vi "coag model linear regression.vi"(4 "averaged data":T1, 6 "all coag in":dbl[](array[numeric]), 7 "scans":i32, 9 "target clarified turbidity (NTU)":dbl, 10 "dose updates per HRT":u32, 11 "all data in":T1[](array[typedef])) -> (1 "coag dose":dbl, 2 "Ccoag-DOM":dbl, 3 "Graph":cluster{dbl[], "Best Linear Fit":dbl[]}[](array[cluster]), 5 "Ku*":dbl)   [LabVIEW 2015]
uses:
  <vilib>/Analysis/NI_AALPro.lvlib
  data cluster.ctl
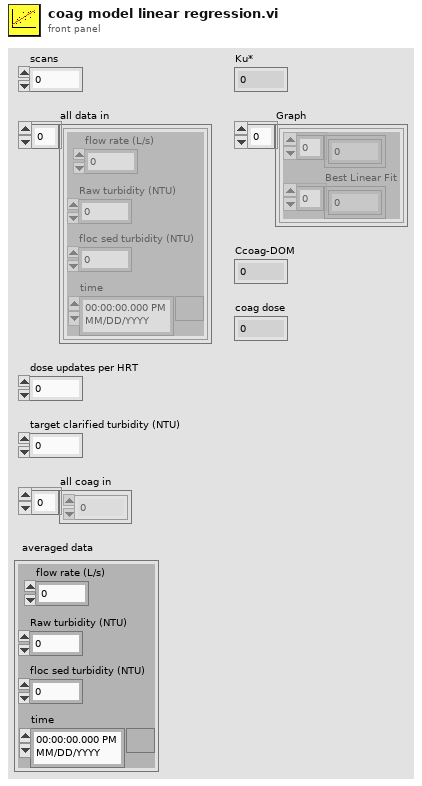
[diagram p1: front panel]
types:
  T1 = typedef "data cluster.ctl" = cluster{"floc sed turbidity (NTU)":dbl, "Raw turbidity (NTU)":dbl, "flow rate (L/s)":dbl, "time":timestamp}
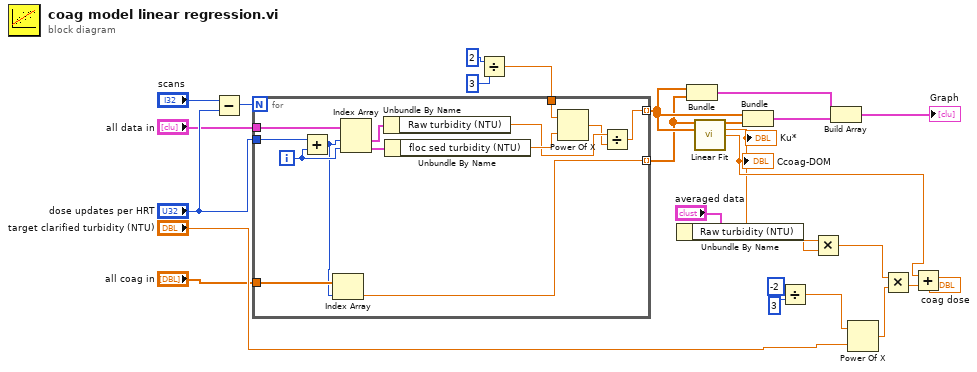
[diagram p0: block diagram]
diagram:
  n1 = Subtract(x="scans", y="dose updates per HRT") -> (x-y=w2:u32)
  n2 = Divide(x=2, y=3) -> (x/y=w6:dbl)
  n3 = for {
    N: w2 -> [_]
    tunnel: "all data in" -> [w39]
    tunnel: "dose updates per HRT" -> [w38]
    tunnel: w6 -> [w34]
    tunnel: "all coag in" -> [w30]
    tunnel: [w28] -> w9 mode=indexing
    tunnel: [w27] -> w8 mode=indexing
    i -> [w37]
    n4 = Add(x=w38, y=w37) -> (x+y=w29:u32)
    n5 = Index Array(array=w30, index=w29) -> (element=w27:dbl)
    n6 = Index Array(array=w39, index #1=w29, index #2=w37) -> (element #1=w36:T1, element #2=w35:T1)
    n7 = Unbundle By Name(w36) -> ("Raw turbidity (NTU)"=w32:dbl)
    n8 = Unbundle By Name(w35) -> ("floc sed turbidity (NTU)"=w33:dbl)
    n9 = Power Of X(1:w33, 2:w34) -> (0:w31:dbl)
    n10 = Divide(x=w32, y=w31) -> (x/y=w28:dbl)
  }
  n11 = Unbundle By Name("averaged data") -> ("Raw turbidity (NTU)"=w20:dbl)
  n12 = Bundle(w9, w8) -> (w11:cluster{dbl[], dbl[]})  [unwired: 1 in]
  n13 = call <vilib>:"Linear Fit.vi"("Y"=w8, "X"=w9) -> ("Best Linear Fit"=w10:dbl[], "slope"=w21:dbl, "intercept"=w24:dbl)  [unwired: 9 in, 2 out]
  "Ku*" <- w21
  "Ccoag-DOM" <- w24
  n14 = Bundle(w9, "Best Linear Fit"=w10) -> (w12:cluster{dbl[], "Best Linear Fit":dbl[]})  [unwired: 1 in]
  n15 = Divide(x=-2, y=3) -> (x/y=w16:dbl)
  n16 = Multiply(x=w21, y=w20) -> (x*y=w17:dbl)
  n17 = Build Array(w11, w12) -> (→"Graph":cluster{dbl[], "Best Linear Fit":dbl[]}[])
  n18 = Power Of X(1:"target clarified turbidity (NTU)", 2:w16) -> (0:w18:dbl)
  n19 = Multiply(x=w17, y=w18) -> (x*y=w23:dbl)
  n20 = Add(x=w24, y=w23) -> (x+y=→"coag dose":dbl)
